vi "Run_EnFlo_Hub.vi"(4 "Error In":errorcluster) -> (0 "Error Out":errorcluster)   [LabVIEW 2020]
panel:
  out "whoCalledMe":string
  out "No of iterations":i32
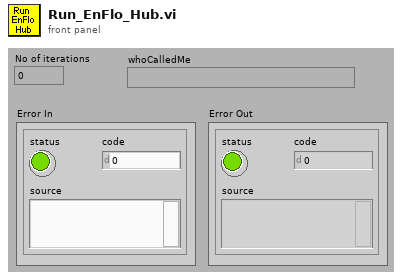
[diagram p1: front panel]
types:
  T1 = enum32{"Bad", "Idle", "Run top level", "Running"}
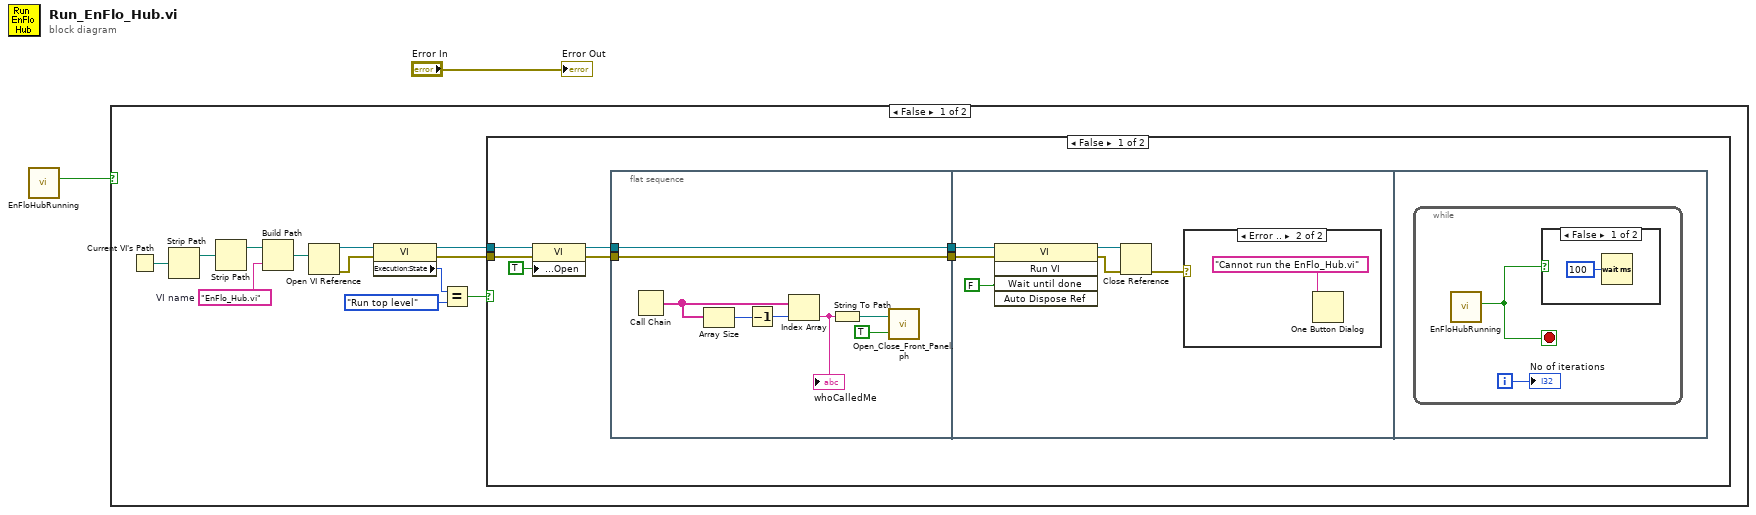
[diagram p0: block diagram]
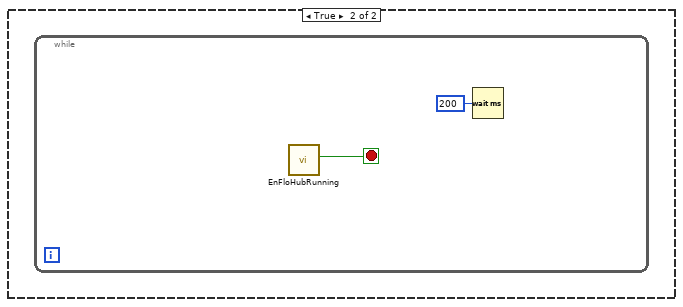
[diagram p4: hidden frame]
diagram:
  n1 = call "EnFloHubRunning.vi"() -> ("EnFloHubRunning"=w1:bool)  [unwired: 11 in]
  n2 = case shown="False" w1 {
    frame False {
      w9 = "EnFlo_Hub.vi"  # VI name
      n3 = Current VI's Path() -> (path=w8:path)
      n4 = Strip Path(path=w8) -> (stripped path=w10:path)  [unwired: 1 out]
      n5 = Strip Path(path=w10) -> (stripped path=w11:path)  [unwired: 1 out]
      n6 = Build Path(base path=w11, name or relative path=w9) -> (appended path=w14:path)
      n7 = Open VI Reference(vi path=w14) -> (vi reference=w12:refnum<vi>, error out=w13:errorcluster)  [unwired: 2 in, 3 out]
      n8 = property class="VI"(reference=w12, error in=w13) -> (reference out=w3:refnum<vi>, error out=w4:errorcluster, "Execution:State"=w7:T1)
      n9 = Equal?(x=w7, y=T1."Run top level" ("Execution:State")) -> (x = y?=w5:bool)
      n10 = case shown="False" w5 {
        tunnel: w4 -> [w20 _]
        tunnel: w3 -> [w19 _]
        frame False {
          n11 = property class="VI"(reference=w19, error in=w20, "Front Panel Window:Open"=TRUE) -> (reference out=w18:refnum<vi>, error out=w17:errorcluster)
          n12 = flat-sequence {
            tunnel: w18 -> [w23]
            tunnel: [w23] -> w16
            tunnel: w17 -> [w22]
            tunnel: [w22] -> w15
            tunnel: w16 -> [w31]
            tunnel: w15 -> [w30]
            frame #0 {
              n13 = Call Chain() -> (call chain=w24:string[])
              n14 = Array Size(array=w24) -> (size(s)=w29:i32)
              n15 = Decrement(x=w29) -> (x-1=w28:i32)
              n16 = Index Array(array=w24, index=w28) -> (element=w27:string)
              "whoCalledMe" <- w27
              n17 = String To Path(string=w27) -> (path=w26:path)
              n18 = call "Open_Close_Front_Panel.ph.vi"("openWindow (T)"=TRUE ("Front Panel Window:Open"), "VI path"=w26) -> ()  [unwired: 2 out]
            }
            frame #1 {
              w35 = FALSE ("Wait until done")
              n19 = invoke class="VI" method="Run VI"(reference=w31, error in=w30, "Wait until done"=w35, "Auto Dispose Ref"=w35) -> (reference out=w34:refnum<vi>, error out=w33:errorcluster)  [unwired: 1 in, 3 out]
              n20 = Close Reference(reference=w34, error in (no error)=w33) -> (error out=w32:errorcluster)
              n21 = case shown="Error .." w32 {
                frame No Error {
                }
                frame Error {
                  n22 = One Button Dialog(message="Cannot run the EnFlo_Hub.vi") -> ()  [unwired: 2 out]
                }
              }
            }
            frame #2 {
              n23 = while {
                i -> [w38]
                stop <- w37 stop-if-true
                n24 = call "EnFloHubRunning.vi"() -> ("EnFloHubRunning"=w37:bool)  [unwired: 11 in]
                n25 = case shown="False" w37 {
                  frame False {
                    n26 = Wait (ms)(milliseconds to wait=u32 100) -> ()  [unwired: 1 out]
                  }
                  frame True {
                  }
                }
                "No of iterations" <- w38
              }
            }
          }
        }
        frame True {
          n27 = while {
            stop <- w40 stop-if-true
            n28 = call "EnFloHubRunning.vi"() -> ("EnFloHubRunning"=w40:bool)  [unwired: 11 in]
            n29 = Wait (ms)(milliseconds to wait=u32 200) -> ()  [unwired: 1 out]
          }
        }
      }
    }
    frame True {
    }
  }
  "Error Out" <- "Error In"
